vi "Subscribe API to Test Runner.vi"(8 "error in (no error)":errorcluster, 11 "Execution API In":refnum<class "Execution API.lvclass">) -> (0 "error out":errorcluster, 3 "Execution API Out":refnum<class "Execution API.lvclass">)   [LabVIEW 2020, in "Execution API.lvclass"]
uses:
  Execution API.lvclass
  C:/git/astemes-lunit/source/Framework/Result Observer/Result Observer.lvclass
  Execution API.lvclass/Execution API.ctl
  Framework/Test Runner/Test Runner.lvclass
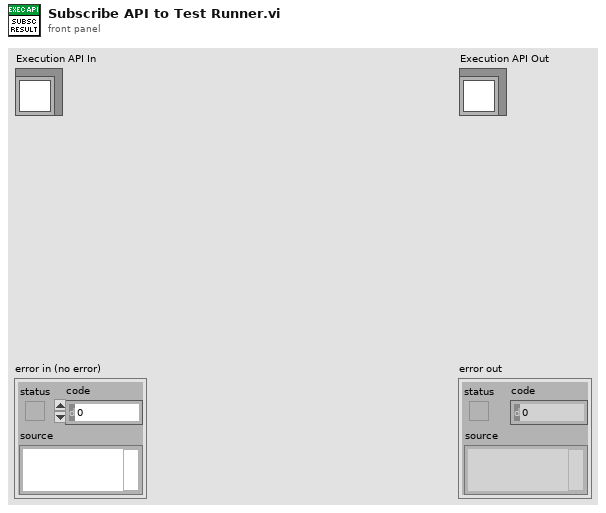
[diagram p1: front panel]
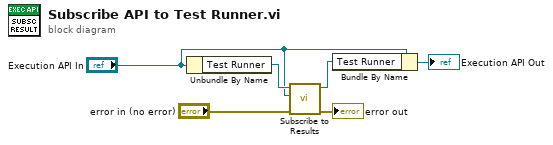
[diagram p0: block diagram]
diagram:
  n1 = Unbundle By Name("Execution API In") -> ("Test Runner"=w6:refnum<class "Test Runner.lvclass">)
  n2 = call-dynamic "Subscribe to Results.vi"("error in (no error)"="error in (no error)", "Result Observer"="Execution API In", "Test Runner In"=w6) -> ("error out"=→"error out":errorcluster, "Test Runner Out"=w3:refnum<class "Test Runner.lvclass">)  [unwired: 7 in]
  n3 = Bundle By Name(cluster="Execution API In", "Test Runner"=w3) -> (→"Execution API Out":refnum<class "Execution API.lvclass">)
